vi "List Child Fields.vi"(7 "field name":string, 8 "error in (no error)":errorcluster, 11 "PV Data in":refnum<class "PV Data.lvclass">) -> (0 "error out":errorcluster, 2 "field names":string[](array[string]), 3 "PV Data out":refnum<class "PV Data.lvclass">)   [LabVIEW 2020, in "PV Access.lvlib" / "PV Data.lvlib" / "PV Data.lvclass"]
uses:
  PV Data.lvclass
  PV Data.lvclass/PV Data.ctl
  PV Access.lvlib
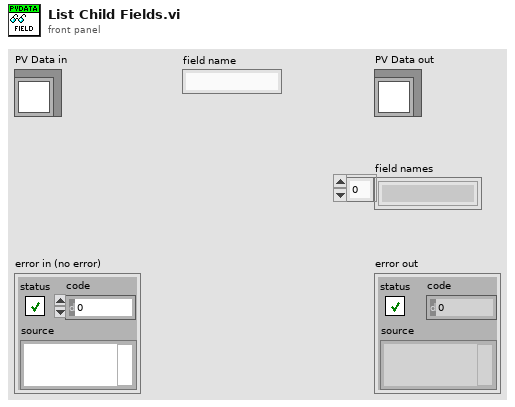
[diagram p1: front panel]
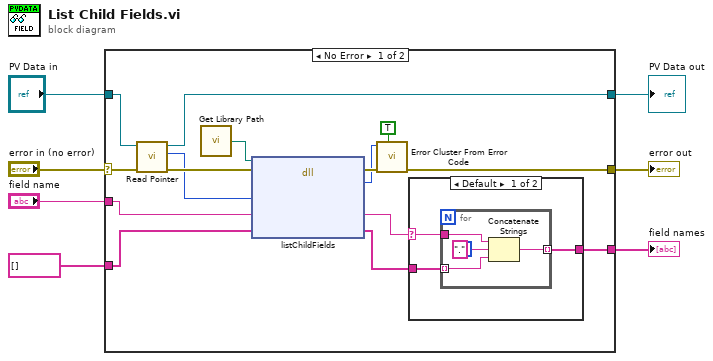
[diagram p0: block diagram]
diagram:
  n1 = case shown="No Error" "error in (no error)" {
    selector: "error in (no error)" -> [w17 w33]
    tunnel: [w18 w33] -> w7
    tunnel: "PV Data in" -> [w15 w32]
    tunnel: [w13 w32] -> w4
    tunnel: string[] [] ("value") -> [w12 w31]
    tunnel: [w8 w31] -> w2
    tunnel: "field name" -> [w11 _]
    frame No Error {
      n2 = call-dynamic "Read Pointer.vi"("error in (no error)"=w17, "Pointer Base in"=w15) -> ("error out"=w16:errorcluster, "Pointer"=w14:i64, "Pointer Base out"=w13:refnum<class "PV Data.lvclass">)  [unwired: 7 in]
      n3 = call "Get Library Path.vi"() -> ("Path"=w22:path)  [unwired: 1 in]
      n4 = dll-call lib="?" fn="listChildFields"(path in=w22, error in=w16, "value"=w14, "field_name"=w11, "child_field_names"=w12) -> (error out=w20:errorcluster, "err_code"=w19:i32, "field_name"=w10:string, "child_field_names"=w9:string[])  [unwired: 2 in, 1 out]
      n5 = call <vilib>:"Error Cluster From Error Code.vi"("show call chain? (False)"=TRUE, "error in (no error)"=w20, "error code (0)"=w19) -> ("error out"=w18:errorcluster)  [unwired: 6 in]
      n6 = case shown="Default" w10 {
        selector: w10 -> [w23 _]
        tunnel: [w24 w30] -> w8
        tunnel: w9 -> [w25 w30]
        frame Default {
          n7 = for {
            tunnel: w25 -> [w29] mode=indexing
            tunnel: [w28] -> w24 mode=indexing
            tunnel: w23 -> [w26]
            n8 = Concatenate Strings(w26, ".", w29) -> (w28:string)
          }
        }
        frame "" {
        }
      }
    }
    frame Error {
    }
  }
  "error out" <- w7
  "field names" <- w2
  "PV Data out" <- w4
